vi "PinholesRolling.vi"(4 "Current Threshold [nA]":dbl, 5 "settling\ndelay":i32, 6 "Probe Card Channels":i32=32) -> (0 "Compliance?":bool, 1 "excluded channels":i32[](array[numeric]), 2 "Current [nA]":dbl[](array[numeric]), 3 "Flag":i32[](array[numeric]))   [LabVIEW 2013]
uses:
  InstrControl/ProbeStationControl/ProbeStationControl.lvclass
  general_VIs/globals/QC_MeasurementSetup.vi
  InstrControl/InstrumentSetup.vi
  InstrControl/SupplyControl/SupplyControl.lvclass
  InstrControl/Switching/Switching.lvclass
  InstrControl/InstrControl.lvclass
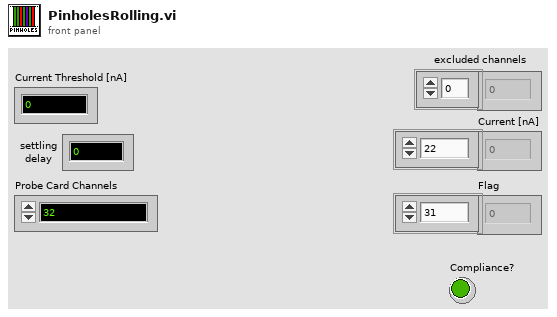
[diagram p1: front panel]
types:
  T1 = enum16{"Reference measurement", "Baseline correcetion 10V", "Baseline correcetion 100V", "Nothing"}
  T2 = cluster{"Bias Supply":refnum<class "SupplyControl.lvclass">, "SMU":refnum<class "SupplyControl.lvclass">, "LCR":refnum<class "LCRControl.lvclass">, "Probe Card Channels":i32, "Bias Voltage [V]":dbl, "First strip":i32, "Last strip":i32, "Base Voltage [V]":dbl, "Base Ramp Step [V]":dbl, "Base Ramp Interval [ms]":u32, "High Voltage [V]":dbl, "High Ramp Step [V]":dbl, "High Ramp Interval [ms]":u32, "Single Needle":bool, "ArduinoControl.lvclass":refnum<class "ArduinoControl.lvclass">, "Fraction of good strips [%]":dbl}
  T3 = cluster{"GPIB address":string, "Matrix address":string, "Mux1 address":string, "Mux2 address":string, "Matrix used?":bool, "Switching":refnum<class "Switching.lvclass">, "Matrix X Channels":cluster{"Bias Supply / SMU LO":i32, "Bias Supply / SMU HI":i32, "CV Box LO":i32, "CV Box HI":i32, "CV Box LO IN":i32, "CV Box HI IN":i32, "Volt meter LO":i32, "Volt meter HI":i32, "Mux1 C1":i32, "Mux1 C2":i32, "Mux2 C1":i32, "Mux2 C2":i32}}
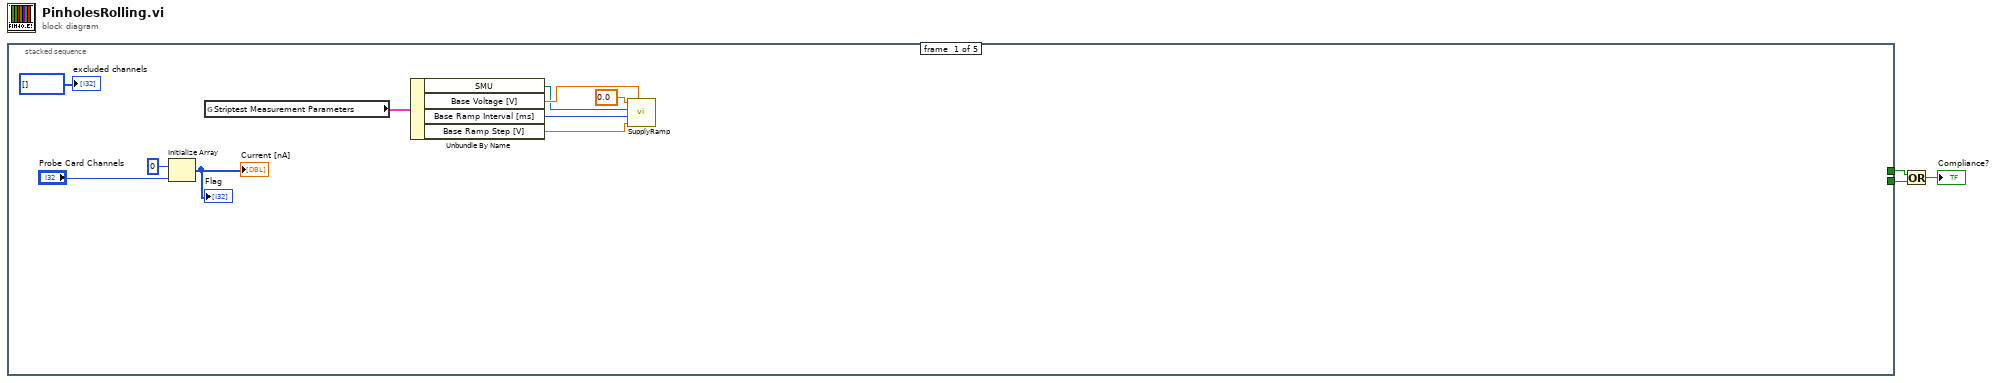
[diagram p0: block diagram]
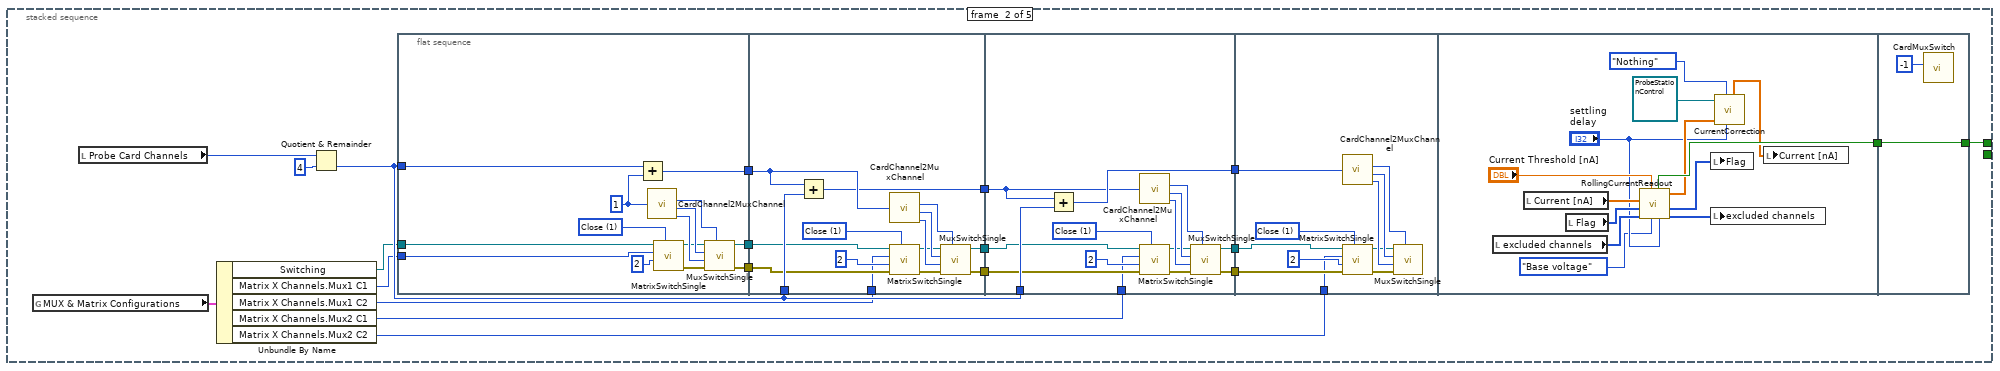
[diagram p2: hidden frame]
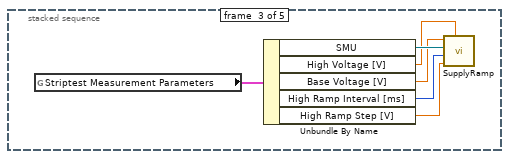
[diagram p3: hidden frame]
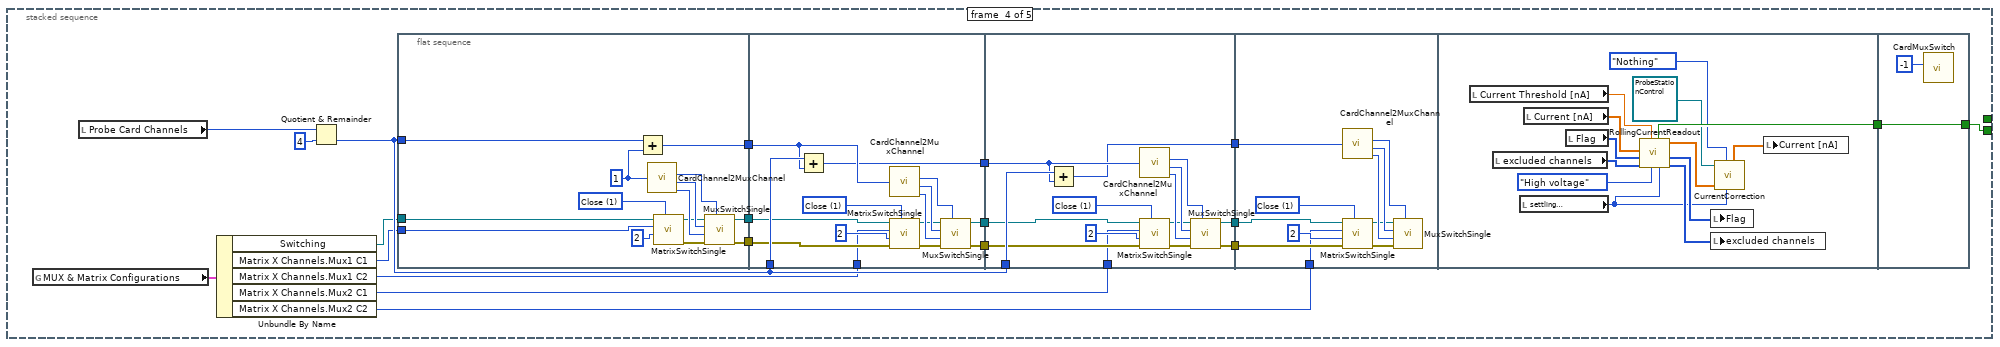
[diagram p4: hidden frame]
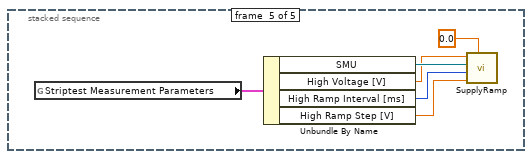
[diagram p5: hidden frame]
diagram:
  n1 = stacked-sequence {
    tunnel: [_ _ _ w110 _] -> w2
    tunnel: [_ w14 _ _ _] -> w1
    frame #0 {
      n2 = Initialize Array(0, "Probe Card Channels") -> (→"Flag" →"Current [nA]":i32[])
      n3 = global read "QC_MeasurementSetup.vi" "Striptest Measurement Parameters"() -> (w8:T2)
      n4 = Unbundle By Name(w8) -> ("SMU"=w4:refnum<class "SupplyControl.lvclass">, "Base Voltage [V]"=w7:dbl, "Base Ramp Interval [ms]"=w6:u32, "Base Ramp Step [V]"=w5:dbl)
      n5 = call "SupplyRamp.vi"("Requested Voltage"=w7, "Step Size"=w5, "Step Delay"=w6, "Supply IN"=w4, "Starting Voltage"=0.0) -> ()  [unwired: 3 in, 4 out]
      "excluded channels" <- i32[] []
    }
    frame #1 {
      n6 = global read "InstrumentSetup.vi" "MUX & Matrix Configurations"() -> (w20:T3)
      n7 = local read "Probe Card Channels"() -> (w32:i32)
      n8 = Unbundle By Name(w20) -> ("Switching"=w15:refnum<class "Switching.lvclass">, "Matrix X Channels.Mux1 C1"=w19:i32, "Matrix X Channels.Mux1 C2"=w18:i32, "Matrix X Channels.Mux2 C1"=w17:i32, "Matrix X Channels.Mux2 C2"=w16:i32)
      n9 = Quotient & Remainder(x=w32, y=4) -> (floor(x/y)=w28:i32)  [unwired: 1 out]
      n10 = flat-sequence {
        tunnel: w28 -> [w41]
        tunnel: [w40] -> w30
        tunnel: [w37] -> w26
        tunnel: [w36] -> w25
        tunnel: w19 -> [w35]
        tunnel: w15 -> [w34]
        tunnel: w30 -> [w57]
        tunnel: w28 -> [w56]
        tunnel: [w55] -> w29
        tunnel: w26 -> [w52]
        tunnel: w25 -> [w51]
        tunnel: [w50] -> w24
        tunnel: [w49] -> w23
        tunnel: w18 -> [w48]
        tunnel: w29 -> [w70]
        tunnel: w28 -> [w72]
        tunnel: [w71] -> w27
        tunnel: w24 -> [w67]
        tunnel: w23 -> [w66]
        tunnel: [w65] -> w22
        tunnel: [w64] -> w21
        tunnel: w17 -> [w63]
        tunnel: w27 -> [w83]
        tunnel: w22 -> [w80]
        tunnel: w21 -> [w79]
        tunnel: w16 -> [w78]
        tunnel: [w95] -> w33
        tunnel: [w103] -> w14
        tunnel: w33 -> [w103]
        frame #0 {
          w42 = 1
          w47 = u16 1 items=["Open", "Close"] ("Switch action")
          n11 = Add(x=w41, y=w42) -> (x+y=w40:i32)
          n12 = call "CardChannel2MuxChannel.vi"("Probecard Channel No."=w42) -> ("Mux No.:"=w44:u32, "C1 / C2"=w45:i32, "Channel"=w46:i32)  [unwired: 1 out]
          n13 = call "MatrixSwitchSingle.vi"("Switch action"=w47, "Matrix Y"=2, "Matrix X"=w35, "Switching in"=w34) -> ("error out"=w38:errorcluster, "Switching out"=w39:refnum<class "Switching.lvclass">)  [unwired: 5 in, 1 out]
          n14 = call "MuxSwitchSingle.vi"("MUX address"=w44, "error in (no error)"=w38, "Channel"=w46, "C1 / C2"=w45, "Switching in"=w39) -> ("error out"=w36:errorcluster, "Switching out"=w37:refnum<class "Switching.lvclass">)  [unwired: 4 in, 1 out]
        }
        frame #1 {
          w59 = u16 1 items=["Open", "Close"] ("Switch action")
          n15 = Add(x=w57, y=w56) -> (x+y=w55:i32)
          n16 = call "CardChannel2MuxChannel.vi"("Probecard Channel No."=w57) -> ("Mux No.:"=w60:u32, "C1 / C2"=w61:i32, "Channel"=w62:i32)  [unwired: 1 out]
          n17 = call "MatrixSwitchSingle.vi"("Switch action"=w59, "error in (no error)"=w51, "Matrix Y"=2, "Matrix X"=w48, "Switching in"=w52) -> ("error out"=w53:errorcluster, "Switching out"=w54:refnum<class "Switching.lvclass">)  [unwired: 4 in, 1 out]
          n18 = call "MuxSwitchSingle.vi"("MUX address"=w60, "error in (no error)"=w53, "Channel"=w62, "C1 / C2"=w61, "Switching in"=w54) -> ("error out"=w49:errorcluster, "Switching out"=w50:refnum<class "Switching.lvclass">)  [unwired: 4 in, 1 out]
        }
        frame #2 {
          w76 = u16 1 items=["Open", "Close"] ("Switch action")
          n19 = Add(x=w70, y=w72) -> (x+y=w71:i32)
          n20 = call "CardChannel2MuxChannel.vi"("Probecard Channel No."=w70) -> ("Mux No.:"=w75:u32, "C1 / C2"=w74:i32, "Channel"=w73:i32)  [unwired: 1 out]
          n21 = call "MatrixSwitchSingle.vi"("Switch action"=w76, "error in (no error)"=w66, "Matrix Y"=2, "Matrix X"=w63, "Switching in"=w67) -> ("error out"=w69:errorcluster, "Switching out"=w68:refnum<class "Switching.lvclass">)  [unwired: 4 in, 1 out]
          n22 = call "MuxSwitchSingle.vi"("MUX address"=w75, "error in (no error)"=w69, "Channel"=w73, "C1 / C2"=w74, "Switching in"=w68) -> ("error out"=w64:errorcluster, "Switching out"=w65:refnum<class "Switching.lvclass">)  [unwired: 4 in, 1 out]
        }
        frame #3 {
          w85 = u16 1 items=["Open", "Close"] ("Switch action")
          n23 = call "CardChannel2MuxChannel.vi"("Probecard Channel No."=w83) -> ("Mux No.:"=w86:u32, "C1 / C2"=w87:i32, "Channel"=w88:i32)  [unwired: 1 out]
          n24 = call "MatrixSwitchSingle.vi"("Switch action"=w85, "error in (no error)"=w79, "Matrix Y"=2, "Matrix X"=w78, "Switching in"=w80) -> ("error out"=w82:errorcluster, "Switching out"=w81:refnum<class "Switching.lvclass">)  [unwired: 4 in, 1 out]
          n25 = call "MuxSwitchSingle.vi"("MUX address"=w86, "error in (no error)"=w82, "Channel"=w88, "C1 / C2"=w87, "Switching in"=w81) -> ()  [unwired: 4 in, 3 out]
        }
        frame #4 {
          n26 = local read "excluded channels"() -> (w99:i32[])
          n27 = local read "Current [nA]"() -> (w100:dbl[])
          n28 = local read "Flag"() -> (w98:i32[])
          n29 = call "RollingCurrentReadout.vi"("settling\ndelay"="settling\ndelay", "Base/High Voltage?"=enum16{"Base voltage", "High voltage"}."Base voltage", "Current Threshold [nA]"="Current Threshold [nA]", "disabled channels IN"=w99, "Flag IN"=w98, "Current Array IN [nA]"=w100) -> ("disabled channels OUT"=w97:i32[], "Flag OUT"=w96:i32[], "Current Array OUT [nA]"=w94:dbl[], "Compliance exceeded"=w95:bool)  [unwired: 2 in]
          n30 = local write "Flag"(w96) -> ()
          n31 = local write "excluded channels"(w97) -> ()
          n32 = call "CurrentCorrection.vi"("ProbeStationControl in"=refnum<class "ProbeStationControl.lvclass"> refnum, "Action"=T1."Nothing", "Current IN"=w94, "settling\ndelay"="settling\ndelay") -> ("Current OUT"=w93:dbl[])  [unwired: 1 in, 4 out]
          n33 = local write "Current [nA]"(w93) -> ()
        }
        frame #5 {
          n34 = call "CardMuxSwitch.vi"("Switch to channel"=-1) -> ()  [unwired: 10 in, 1 out]
        }
      }
    }
    frame #2 {
      n35 = global read "QC_MeasurementSetup.vi" "Striptest Measurement Parameters"() -> (w109:T2)
      n36 = Unbundle By Name(w109) -> ("SMU"=w106:refnum<class "SupplyControl.lvclass">, "High Voltage [V]"=w104:dbl, "Base Voltage [V]"=w105:dbl, "High Ramp Interval [ms]"=w107:u32, "High Ramp Step [V]"=w108:dbl)
      n37 = call "SupplyRamp.vi"("Requested Voltage"=w104, "Step Size"=w108, "Step Delay"=w107, "Supply IN"=w106, "Starting Voltage"=w105) -> ()  [unwired: 3 in, 4 out]
    }
    frame #3 {
      n38 = global read "InstrumentSetup.vi" "MUX & Matrix Configurations"() -> (w116:T3)
      n39 = local read "Probe Card Channels"() -> (w128:i32)
      n40 = Unbundle By Name(w116) -> ("Switching"=w115:refnum<class "Switching.lvclass">, "Matrix X Channels.Mux1 C1"=w114:i32, "Matrix X Channels.Mux1 C2"=w113:i32, "Matrix X Channels.Mux2 C1"=w112:i32, "Matrix X Channels.Mux2 C2"=w111:i32)
      n41 = Quotient & Remainder(x=w128, y=4) -> (floor(x/y)=w126:i32)  [unwired: 1 out]
      n42 = flat-sequence {
        tunnel: w126 -> [w138]
        tunnel: [w136] -> w125
        tunnel: [w133] -> w122
        tunnel: [w132] -> w121
        tunnel: w115 -> [w131]
        tunnel: w114 -> [w130]
        tunnel: w126 -> [w153]
        tunnel: w125 -> [w152]
        tunnel: [w151] -> w124
        tunnel: w122 -> [w150]
        tunnel: w121 -> [w147]
        tunnel: [w146] -> w120
        tunnel: [w145] -> w119
        tunnel: w113 -> [w144]
        tunnel: w126 -> [w168]
        tunnel: w124 -> [w167]
        tunnel: [w166] -> w123
        tunnel: w120 -> [w165]
        tunnel: w119 -> [w164]
        tunnel: [w161] -> w118
        tunnel: [w160] -> w117
        tunnel: w112 -> [w159]
        tunnel: w123 -> [w179]
        tunnel: w118 -> [w178]
        tunnel: w117 -> [w177]
        tunnel: w111 -> [w174]
        tunnel: [w192] -> w129
        tunnel: [w199] -> w110
        tunnel: w129 -> [w199]
        frame #0 {
          w137 = 1
          w143 = u16 1 items=["Open", "Close"] ("Switch action")
          n43 = Add(x=w138, y=w137) -> (x+y=w136:i32)
          n44 = call "CardChannel2MuxChannel.vi"("Probecard Channel No."=w137) -> ("Mux No.:"=w140:u32, "C1 / C2"=w141:i32, "Channel"=w142:i32)  [unwired: 1 out]
          n45 = call "MatrixSwitchSingle.vi"("Switch action"=w143, "Matrix Y"=2, "Matrix X"=w130, "Switching in"=w131) -> ("error out"=w134:errorcluster, "Switching out"=w135:refnum<class "Switching.lvclass">)  [unwired: 5 in, 1 out]
          n46 = call "MuxSwitchSingle.vi"("MUX address"=w140, "error in (no error)"=w134, "Channel"=w142, "C1 / C2"=w141, "Switching in"=w135) -> ("error out"=w133:errorcluster, "Switching out"=w132:refnum<class "Switching.lvclass">)  [unwired: 4 in, 1 out]
        }
        frame #1 {
          w155 = u16 1 items=["Open", "Close"] ("Switch action")
          n47 = Add(x=w153, y=w152) -> (x+y=w151:i32)
          n48 = call "CardChannel2MuxChannel.vi"("Probecard Channel No."=w152) -> ("Mux No.:"=w156:u32, "C1 / C2"=w157:i32, "Channel"=w158:i32)  [unwired: 1 out]
          n49 = call "MatrixSwitchSingle.vi"("Switch action"=w155, "error in (no error)"=w150, "Matrix Y"=2, "Matrix X"=w144, "Switching in"=w147) -> ("error out"=w148:errorcluster, "Switching out"=w149:refnum<class "Switching.lvclass">)  [unwired: 4 in, 1 out]
          n50 = call "MuxSwitchSingle.vi"("MUX address"=w156, "error in (no error)"=w148, "Channel"=w158, "C1 / C2"=w157, "Switching in"=w149) -> ("error out"=w145:errorcluster, "Switching out"=w146:refnum<class "Switching.lvclass">)  [unwired: 4 in, 1 out]
        }
        frame #2 {
          w172 = u16 1 items=["Open", "Close"] ("Switch action")
          n51 = Add(x=w168, y=w167) -> (x+y=w166:i32)
          n52 = call "CardChannel2MuxChannel.vi"("Probecard Channel No."=w167) -> ("Mux No.:"=w171:u32, "C1 / C2"=w170:i32, "Channel"=w169:i32)  [unwired: 1 out]
          n53 = call "MatrixSwitchSingle.vi"("Switch action"=w172, "error in (no error)"=w164, "Matrix Y"=2, "Matrix X"=w159, "Switching in"=w165) -> ("error out"=w163:errorcluster, "Switching out"=w162:refnum<class "Switching.lvclass">)  [unwired: 4 in, 1 out]
          n54 = call "MuxSwitchSingle.vi"("MUX address"=w171, "error in (no error)"=w163, "Channel"=w169, "C1 / C2"=w170, "Switching in"=w162) -> ("error out"=w160:errorcluster, "Switching out"=w161:refnum<class "Switching.lvclass">)  [unwired: 4 in, 1 out]
        }
        frame #3 {
          w181 = u16 1 items=["Open", "Close"] ("Switch action")
          n55 = call "CardChannel2MuxChannel.vi"("Probecard Channel No."=w179) -> ("Mux No.:"=w182:u32, "C1 / C2"=w183:i32, "Channel"=w184:i32)  [unwired: 1 out]
          n56 = call "MatrixSwitchSingle.vi"("Switch action"=w181, "error in (no error)"=w177, "Matrix Y"=2, "Matrix X"=w174, "Switching in"=w178) -> ("error out"=w175:errorcluster, "Switching out"=w176:refnum<class "Switching.lvclass">)  [unwired: 4 in, 1 out]
          n57 = call "MuxSwitchSingle.vi"("MUX address"=w182, "error in (no error)"=w175, "Channel"=w184, "C1 / C2"=w183, "Switching in"=w176) -> ()  [unwired: 4 in, 3 out]
        }
        frame #4 {
          n58 = local read "Current Threshold [nA]"() -> (w191:dbl)
          n59 = local read "excluded channels"() -> (w196:i32[])
          n60 = local read "settling\ndelay"() -> (w187:i32)
          n61 = local read "Current [nA]"() -> (w197:dbl[])
          n62 = local read "Flag"() -> (w195:i32[])
          n63 = call "RollingCurrentReadout.vi"("settling\ndelay"=w187, "Base/High Voltage?"=enum16{"Base voltage", "High voltage"}."High voltage", "Current Threshold [nA]"=w191, "disabled channels IN"=w196, "Flag IN"=w195, "Current Array IN [nA]"=w197) -> ("disabled channels OUT"=w194:i32[], "Flag OUT"=w193:i32[], "Current Array OUT [nA]"=w190:dbl[], "Compliance exceeded"=w192:bool)  [unwired: 2 in]
          n64 = local write "Flag"(w193) -> ()
          n65 = local write "excluded channels"(w194) -> ()
          n66 = call "CurrentCorrection.vi"("ProbeStationControl in"=refnum<class "ProbeStationControl.lvclass"> refnum, "Action"=T1."Nothing", "Current IN"=w190, "settling\ndelay"=w187) -> ("Current OUT"=w189:dbl[])  [unwired: 1 in, 4 out]
          n67 = local write "Current [nA]"(w189) -> ()
        }
        frame #5 {
          n68 = call "CardMuxSwitch.vi"("Switch to channel"=-1) -> ()  [unwired: 10 in, 1 out]
        }
      }
    }
    frame #4 {
      n69 = global read "QC_MeasurementSetup.vi" "Striptest Measurement Parameters"() -> (w204:T2)
      n70 = Unbundle By Name(w204) -> ("SMU"=w203:refnum<class "SupplyControl.lvclass">, "High Voltage [V]"=w200:dbl, "High Ramp Interval [ms]"=w201:u32, "High Ramp Step [V]"=w202:dbl)
      n71 = call "SupplyRamp.vi"("Requested Voltage"=0.0, "Step Size"=w202, "Step Delay"=w201, "Supply IN"=w203, "Starting Voltage"=w200) -> ()  [unwired: 3 in, 4 out]
    }
  }
  n72 = Or(x=w1, y=w2) -> (x .or. y?=→"Compliance?":bool)
